vi "isSessionStored.vi"(8 "error in":errorcluster, 10 "Client ID":string, 11 "MQTT Server":refnum<class "Server.lvclass">) -> (0 "error out":errorcluster, 1 "Session Present":bool, 2 "Client ID dup":string, 3 "MQTT Server out":refnum<class "Server.lvclass">, 5 "Stored Session":T1 {"PUBREC" format="%016b"})   [LabVIEW 2013, in "MQTT Server.lvlib" / "Server.lvclass"]
uses:
  Server.lvclass
  StoredSessions/Session State -- cluster.ctl
  <vilib>/LabVIEW Open Source Project/MQTT Control Packets/Control Packets/SUBSCRIBE/Topic Subscription -- cluster.ctl
  <vilib>/LabVIEW Open Source Project/MQTT Control Packets/Control Packets/ControlPacket/QualityOfService -- enum.ctl
  StoredSessions/StoredSessions.lvclass
  <vilib>/LabVIEW Open Source Project/MQTT Control Packets/Control Packets/ControlPacket/ControlPacket.lvclass
  <vilib>/LabVIEW Open Source Project/MQTT Control Packets/Control Packets/SUBSCRIBE/SUBSCRIBE.lvclass
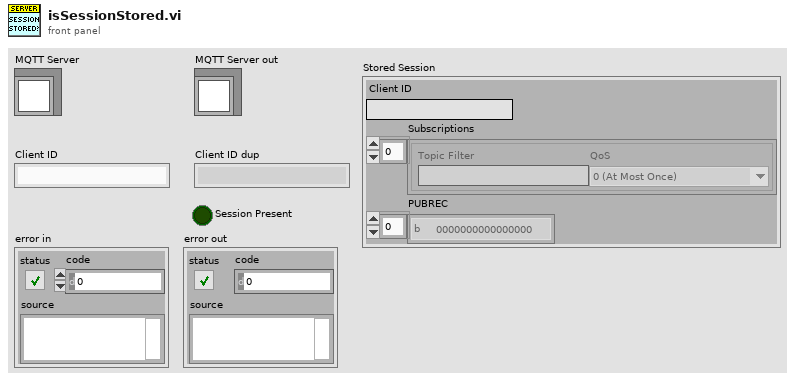
[diagram p1: front panel]
types:
  T1 = typedef "MQTT Server.lvlib/StoredSessions.lvclass/Session State -- cluster.ctl" = cluster{"Client ID":string, "Subscriptions":T2[], "PUBREC":u16[]}
  T2 = typedef "MQTT_Control_Packets.lvlib/SUBSCRIBE.lvclass/Topic Subscription -- cluster.ctl" = cluster{"Topic Filter":string, "QoS":T3}
  T3 = typedef "MQTT_Control_Packets.lvlib/ControlPacket.lvclass/QualityOfService -- enum.ctl" = enum16{"0 (At Most Once)", "1 (At Least Once)", "2 (Exactly Once)"}
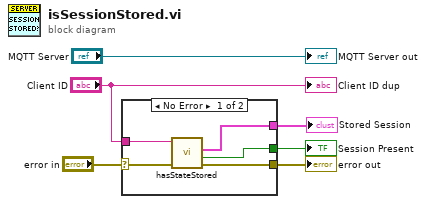
[diagram p0: block diagram]
diagram:
  n1 = case shown="No Error" "error in" {
    selector: "error in" -> [w10 w12]
    tunnel: [w8 w12] -> w5
    tunnel: "Client ID" -> [w11 _]
    tunnel: [w9 _] -> w4
    tunnel: [w7 _] -> w1
    frame No Error {
      n2 = call "hasStateStored.vi"("error in (no error)"=w10, "Client ID"=w11) -> ("error out"=w8:errorcluster, "Found?"=w9:bool, "Stored Session"=w7:T1)  [unwired: 7 in]
    }
    frame Error {
    }
  }
  "error out" <- w5
  "Session Present" <- w4
  "Stored Session" <- w1
  "Client ID dup" <- "Client ID"
  "MQTT Server out" <- "MQTT Server"
